vi "update.vi"(0 "reference in":refnum<class "Observer.lvclass">, 2 "WeatherData":T1, 5 "error in (no error)":errorcluster) -> (14 "reference out":refnum<class "Observer.lvclass">, 19 "error out":errorcluster)   [LabVIEW 2010, in "Observer.lvclass"]
uses:
  Observer.lvclass
  WeatherData.ctl
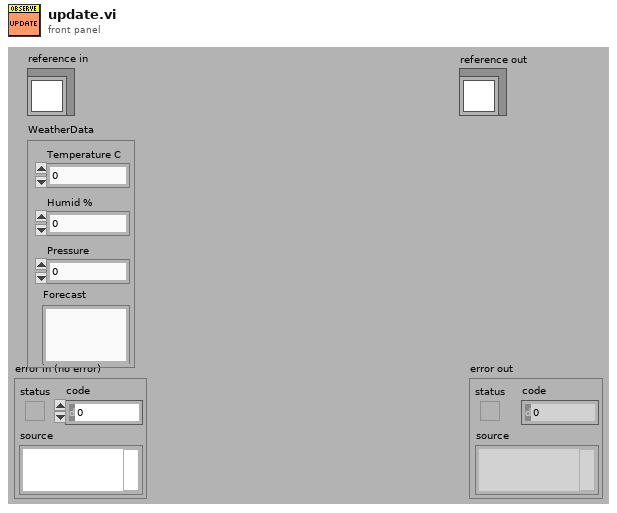
[diagram p1: front panel]
types:
  T1 = typedef "WeatherData.ctl" = cluster{"Temperature C":dbl, "Humid %":dbl, "Pressure":dbl, "Forecast":string}
  T2 = typedef "Observer.lvclass/ObjectAttributes.ctl" = cluster{"Attribute1":dbl}
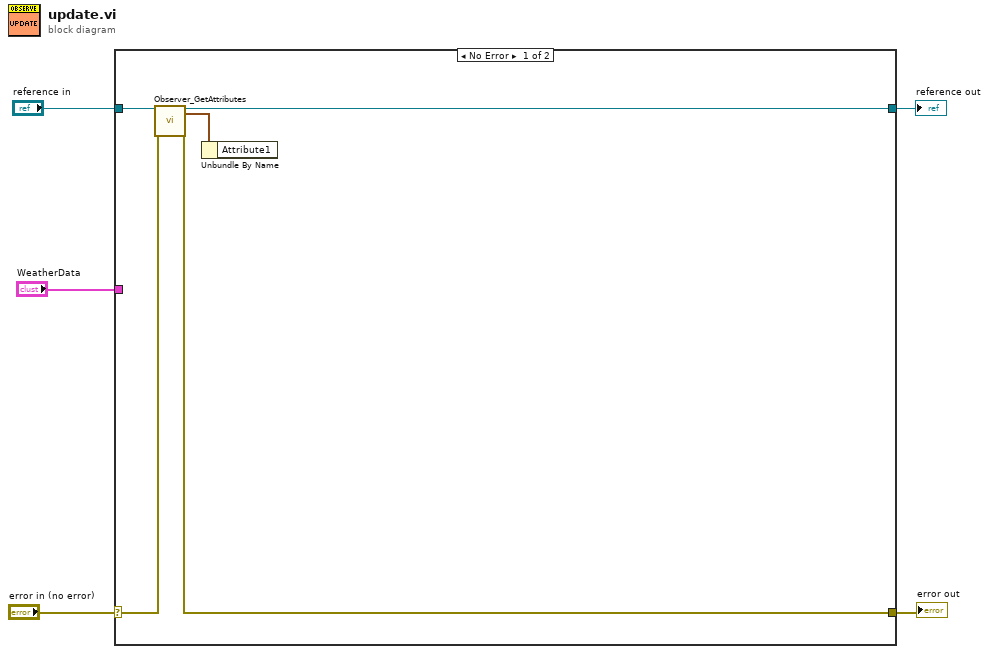
[diagram p0: block diagram]
diagram:
  n1 = case shown="No Error" "error in (no error)" {
    selector: "error in (no error)" -> [w10 w12]
    tunnel: [w8 w12] -> w4
    tunnel: [w6 w11] -> w2
    tunnel: "reference in" -> [w7 w11]
    tunnel: "WeatherData" -> [_ _]
    frame No Error {
      n2 = call "Observer_GetAttributes.vi"("reference in"=w7, "error in (no error)"=w10) -> ("reference out"=w6:refnum<class "Observer.lvclass">, "Data"=w9:T2, "error out"=w8:errorcluster)  [unwired: 14 in, 1 out]
      n3 = Unbundle By Name(w9) -> ()  [unwired: 1 out]
    }
    frame Error {
    }
  }
  "error out" <- w4
  "reference out" <- w2
